vi "SG_calculation.vi"(8 "Error In":errorcluster, 11 "Data":dbl[][](array[numeric])) -> (0 "Error out":errorcluster, 2 "Spectrum":waveform(dbl)[](array[waveform]), 3 "Mean":dbl[](array[numeric]), 4 "ReadyForOutput":bool)   [LabVIEW 2016]
uses:
  MainFGV/MainFGV_mods.ctl
  <vilib>/Analysis/baseanly.llb/Mean (DBL).vi
  <vilib>/Analysis/NI_AALBase.lvlib
  <vilib>/Analysis/NI_AALPro.lvlib
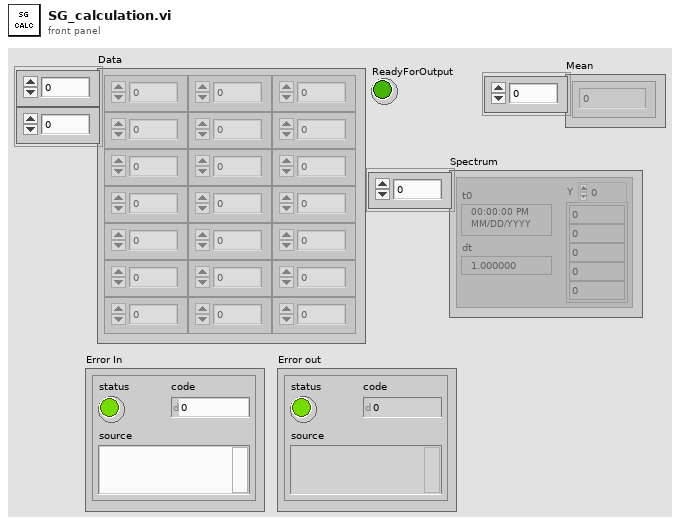
[diagram p1: front panel]
types:
  T1 = typedef "MainFGV_mods.ctl" = enum16{"Init", "Config", "CreateTask", "Register", "Acquire", "Start", "Burst", "Record", "End"}
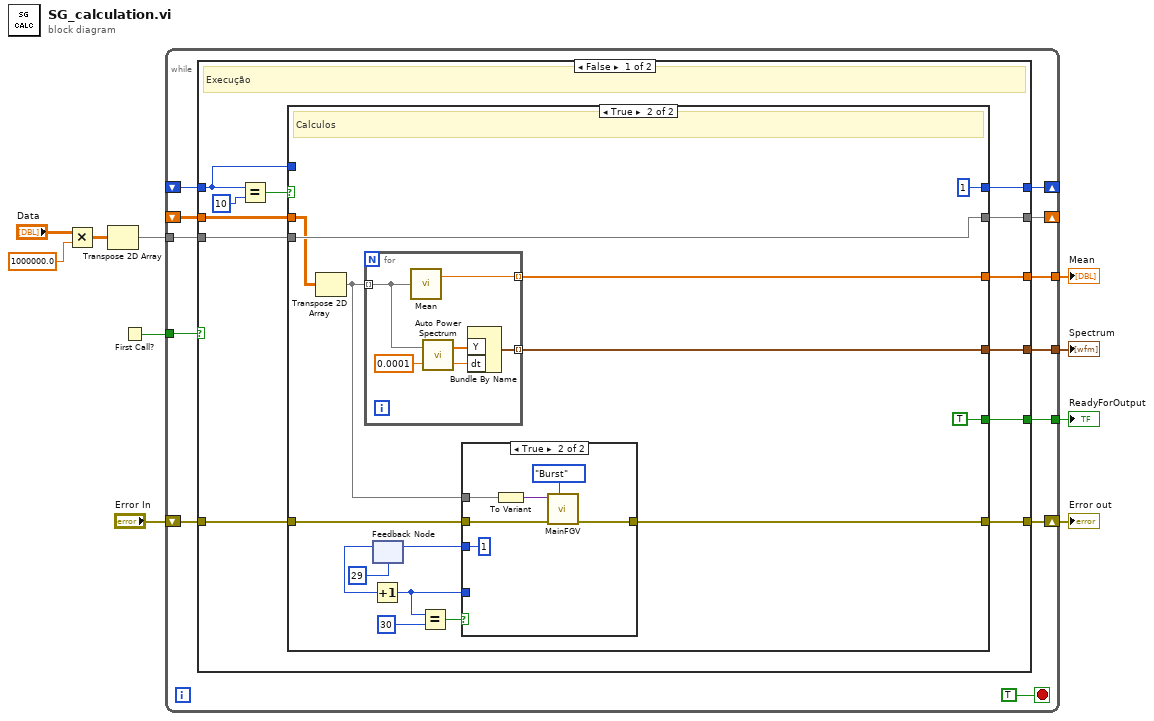
[diagram p0: block diagram]
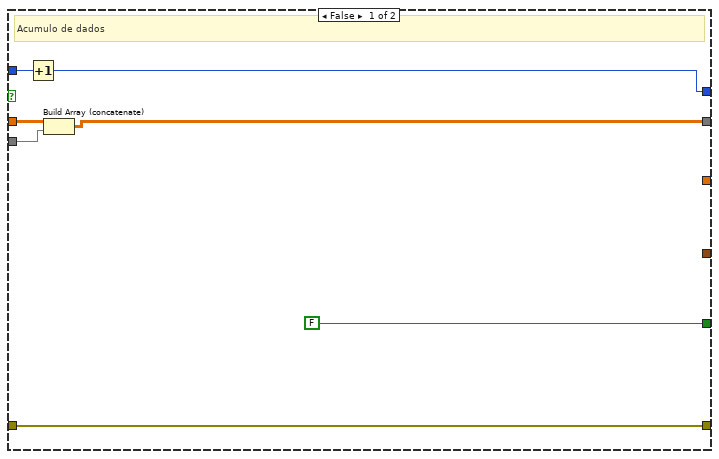
[diagram p2: hidden frame]
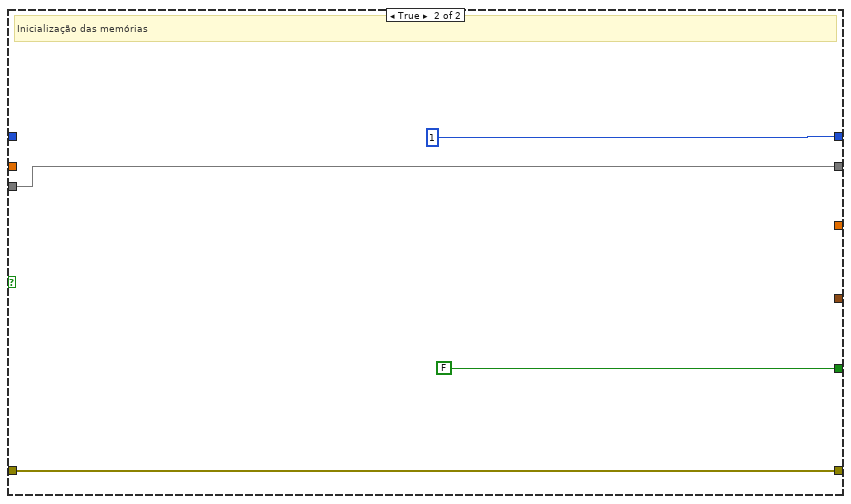
[diagram p4: hidden frame]
diagram:
  n1 = Multiply(x="Data", y=1000000.0) -> (x*y=w5:dbl[][])
  n2 = Transpose 2D Array(2D array=w5) -> (transposed array=w9:dbl[][])
  n3 = First Call?() -> (First Call?: T/F=w10:bool)
  n4 = while {
    tunnel: w9 -> [w20]
    tunnel: w10 -> [w21]
    shift-right: [w19] -> _
    shift-left: _ -> [w16]
    shift-right: [w18] -> _
    shift-left: _ -> [w17]
    tunnel: [w15] -> w8
    tunnel: [w14] -> w7
    tunnel: [w13] -> w3
    shift-right: [w12] -> w1
    shift-left: "Error In" -> [w11]
    stop <- TRUE stop-if-true
    n5 = case shown="False" w21 {
      tunnel: w20 -> [w31 w74]
      tunnel: [w30 w74] -> w19
      tunnel: [w32 1] -> w18
      tunnel: w17 -> [w29 _]
      tunnel: w16 -> [w28 _]
      tunnel: [w27 FALSE] -> w15
      tunnel: [w26 _] -> w14
      tunnel: [w25 _] -> w13
      tunnel: [w24 w71] -> w12
      tunnel: w11 -> [w23 w71]
      frame False {
        # "Execução"
        n6 = Equal?(x=w29, y=10) -> (x = y?=w33:bool)
        n7 = case shown="True" w33 {
          tunnel: [w37 1 ("y")] -> w32
          tunnel: w31 -> [w40 w55]
          tunnel: [w39 w55] -> w30
          tunnel: w28 -> [w41 w53]
          tunnel: w29 -> [w38 _]
          tunnel: [FALSE TRUE] -> w27
          tunnel: [_ w43] -> w26
          tunnel: [_ w42] -> w25
          tunnel: [w35 w45] -> w24
          tunnel: w23 -> [w35 w44]
          frame False {
            # "Acumulo de dados"
            n8 = Increment(x=w38) -> (x+1=w37:i32)
            n9 = Build Array (concatenate)(w41, w40) -> (w39:dbl[][])
          }
          frame True {
            # "Calculos"
            n10 = Transpose 2D Array(2D array=w53) -> (transposed array=w46:dbl[][])
            n11 = for {
              tunnel: w46 -> [w69] mode=indexing
              tunnel: [w70] -> w43 mode=indexing
              tunnel: [w65] -> w42 mode=indexing
              n12 = call-poly <vilib>:"Mean.vi"("X"=w69) -> ("mean"=w70:dbl)  [unwired: 1 out]
              n13 = call <vilib>:"Auto Power Spectrum.vi"("dt"=0.0001, "Signal (V)"=w69) -> ("df"=w66:dbl, "Power Spectrum (V^2 rms)"=w67:dbl[])
              n14 = Bundle By Name("Y"=w67, "dt"=w66) -> (w65:waveform(dbl))  [unwired: 1 in]
            }
            n15 = feedback #1(29 ("y")) -> (w52:i32)
            n16 = Increment(x=w52) -> (x+1=w48:i32)
            n17 = Equal?(x=w48, y=30) -> (x = y?=w49:bool)
            n18 = case shown="True" w49 {
              tunnel: w48 -> [w58 _]
              tunnel: [w58 1] -> w47
              tunnel: w46 -> [_ w63]
              tunnel: [w57 w60] -> w45
              tunnel: w44 -> [w57 w59]
              frame False {
              }
              frame True {
                n19 = To Variant(anything=w63) -> (Variant=w61:variant)
                n20 = call "MainFGV.vi"("FGV_mods"=MainFGV_mods."Burst", "Error In"=w59, "DataIn"=w61) -> ("Error Out"=w60:errorcluster)  [unwired: 7 in, 1 out]
              }
            }
            n21 = feedback-in #1(w47) -> ()
          }
        }
      }
      frame True {
        # "Inicialização das memórias"
      }
    }
  }
  "ReadyForOutput" <- w8
  "Mean" <- w7
  "Spectrum" <- w3
  "Error out" <- w1
